vi "Center Cursor Y.vi"(0 "Display State In":T1, 9 "Container State":T2, 11 "error in (no error)":errorcluster) -> (4 "Display State Out":T1, 15 "error out":errorcluster)   [LabVIEW 2014, in "Graph with cursors XControl.xctl"]
uses:
  Graph with cursors XControl.xctl
  <vilib>/_xctls/Container State.ctl
  Graph with cursors State.ctl
  <vilib>/_xctls/XControlSupport.lvlib
types:
  T1 = typedef "Graph with cursors XControl.xctl/Graph with cursors State.ctl" = cluster{"Cursor names":string[], "Cursor positions":dbl[], "Cursor pairs":i32, "Graph":refnum<vi>, "Prefix":string, "Base path":path}
  T2 = typedef "XControlSupport.lvlib/Container State.ctl" = cluster{"Indicator?":bool, "Run Mode?":bool, " Refnum":refnum<vi>}
  T3 = typedef "LVCursorListTypeDef.ctl" = cluster{"Name":string, "Color":u32, "Style":u8, "Point Style":u8, "Name Visible":bool, "Allow Drag":bool, "Cursor Mode":u32, "Plot":i32, "Index":i32, "Position":cluster{"X":dbl, "Y":dbl}, "X Scale":u32, "Y Scale":u32, "Watch Plots":i32[], "Watch All Plots":bool, "Plot Area":i32, "Label Offset":cluster{"X":dbl, "Y":dbl}}[]
  T4 = cluster{"Name":string, "Color":u32, "Style":u8, "Point Style":u8, "Name Visible":bool, "Allow Drag":bool, "Cursor Mode":u32, "Plot":i32, "Index":i32, "Position":cluster{"X":dbl, "Y":dbl}, "X Scale":u32, "Y Scale":u32, "Watch Plots":i32[], "Watch All Plots":bool, "Plot Area":i32, "Label Offset":cluster{"X":dbl, "Y":dbl}}
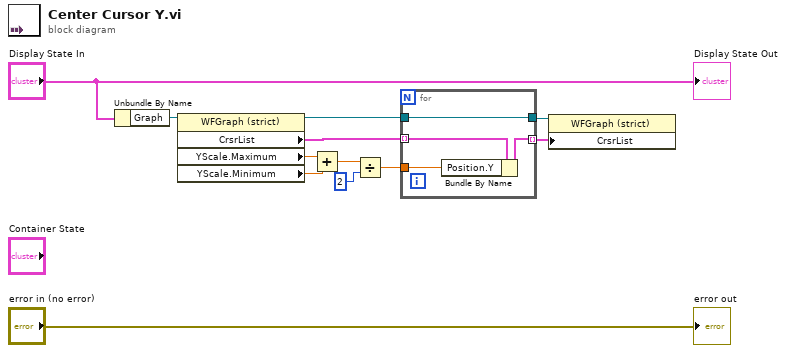
[diagram p0: block diagram]
diagram:
  n1 = Unbundle By Name("Display State In") -> ("Graph"=w11:refnum<vi>)
  n2 = property class="WFGraph (strict)"(reference=w11) -> (reference out=w3:refnum<vi>, "CrsrList"=w5:T3, "YScale.Maximum"=w9:dbl, "YScale.Minimum"=w10:dbl)  [unwired: 1 in, 1 out]
  n3 = Add(x=w9, y=w10) -> (x+y=w8:dbl)
  n4 = Divide(x=w8, y=u32 2) -> (x/y=w6:dbl)
  n5 = for {
    tunnel: w6 -> [w16]
    tunnel: w5 -> [w15] mode=indexing
    tunnel: [w14] -> w1 mode=indexing
    tunnel: [w13] -> w2
    tunnel: w3 -> [w13]
    n6 = Bundle By Name(cluster=w15, "Position.Y"=w16) -> (w14:T4)
  }
  n7 = property class="WFGraph (strict)"(reference=w2, "CrsrList"=w1) -> ()  [unwired: 1 in, 2 out]
  "Display State Out" <- "Display State In"
  "error out" <- "error in (no error)"
